vi "Get ID.vi"() -> (2 "ID":string)   [LabVIEW 2017, in "Example Actor.lvlib" / "Example Actor.lvclass"]
uses:
  Example Actor.lvclass
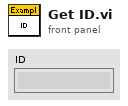
[diagram p1: front panel]
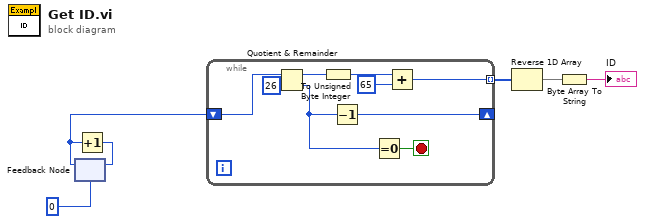
[diagram p0: block diagram]
diagram:
  n1 = feedback #1(0) -> (w1:i32)
  n2 = Increment(x=w1) -> (x+1=w3:i32)
  n3 = feedback-in #1(w3) -> ()
  n4 = while {
    tunnel: [w12] -> w6 mode=indexing
    shift-right: [w7] -> _
    shift-left: w1 -> [w11]
    stop <- w9 stop-if-true
    n5 = Quotient & Remainder(x=w11, y=26) -> (x-y*floor(x/y)=w10:i32, floor(x/y)=w8:i32)
    n6 = To Unsigned Byte Integer(number=w10) -> (unsigned 8bit integer=w13:u8)
    n7 = Decrement(x=w8) -> (x-1=w7:i32)
    n8 = Equal To 0?(x=w8) -> (x = 0?=w9:bool)
    n9 = Add(x=w13, y=u8 65) -> (x+y=w12:u8)
  }
  n10 = Reverse 1D Array(array=w6) -> (reversed array=w4:u8[])
  n11 = Byte Array To String(unsigned byte array=w4) -> (string=→"ID":string)
